vi "GetScanCrvInd.vi"(8 "error in (no error)":errorcluster caption="entrée d'erreur (pas d'erreur)", 10 "Curve Ind":i32, 11 "Interface.lvclass":refnum<class "Interface.lvclass">) -> (0 "error out":errorcluster caption="sortie d'erreur", 2 "Curves Index":i32[](array[numeric]), 3 "Interface.lvclass Out":refnum<class "Interface.lvclass">)   [LabVIEW 2019, in "Interface.lvclass"]
uses:
  Interface.lvclass
  Interface.lvclass/Interface.ctl
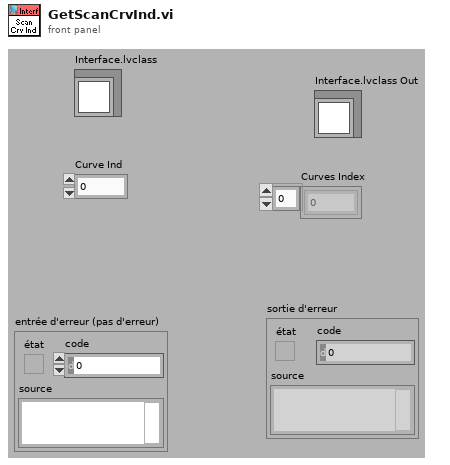
[diagram p1: front panel]
types:
  T1 = typedef "Interface.lvclass/CurveSetup.ctl" = cluster{"CurveName":string, "YParam":string, "XParam":string, "ZParam ":string, "GroupName":string, "LinWdth":u8, "PntCol":u32, "LinCol":u32, "LablFor":u8, "XScale":u32, "YScale":u32, "Interpol":u8, "DisplayName":string, "FillType":i16, "LineStyle":u8, "PntStyle":u8, "BarTyp":u8, "GraphIndex":i32, "Visible":bool, "XScaleName":string, "YScaleName":string, "XYGraph_Ref":refnum<vi>, "Data Only":bool, "DataQ Ref":refnum<queue>, "XParQ Ref":refnum<queue>, "XParamInd":i32, "ScanInd":i32, "File Path":path}
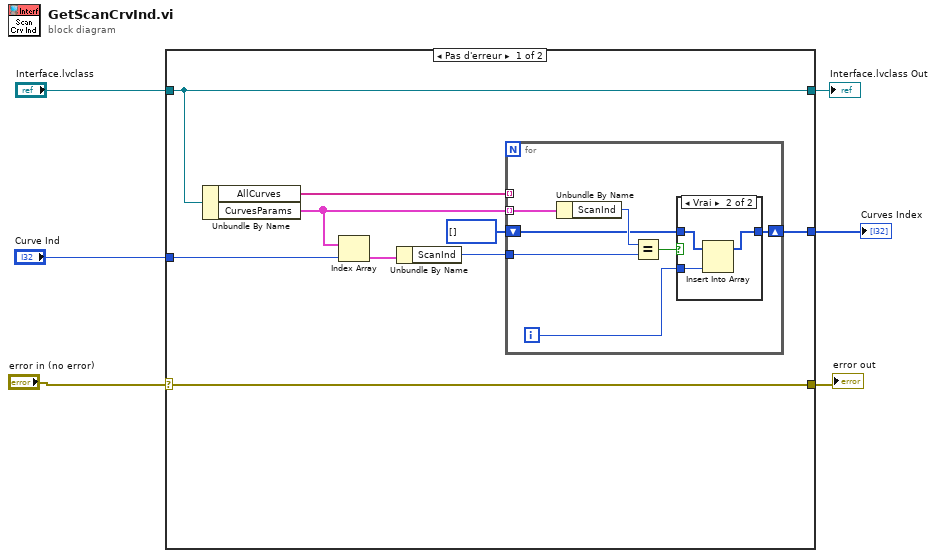
[diagram p0: block diagram]
diagram:
  n1 = case shown="Pas d'erreur" "error in (no error)" {
    selector: "error in (no error)" -> [w15 w28]
    tunnel: [w15 w28] -> w5
    tunnel: [w14 w27] -> w4
    tunnel: "Interface.lvclass" -> [w14 w27]
    tunnel: [w12 _] -> w2
    tunnel: "Curve Ind" -> [w10 _]
    frame No Error {
      n2 = Unbundle By Name(w14) -> ("AllCurves"=w13:string[], "CurvesParams"=w11:T1[])
      n3 = Index Array(array=w11, index=w10) -> (element=w9:T1)
      n4 = Unbundle By Name(w9) -> ("ScanInd"=w8:i32)
      n5 = for {
        tunnel: w13 -> [_] mode=indexing
        tunnel: w11 -> [w22] mode=indexing
        tunnel: w8 -> [w20]
        shift-right: [w17] -> w12
        shift-left: i32[] [] -> [w16]
        i -> [w18]
        n6 = Unbundle By Name(w22) -> ("ScanInd"=w21:i32)
        n7 = Equal?(x=w21, y=w20) -> (x = y?=w19:bool)
        n8 = case shown="Vrai" w19 {
          tunnel: w18 -> [_ w26]
          tunnel: [w23 w25] -> w17
          tunnel: w16 -> [w23 w24]
          frame False {
          }
          frame True {
            n9 = Insert Into Array(array=w24, new element=w26) -> (w25:i32[])  [unwired: 1 in]
          }
        }
      }
    }
    frame Error {
    }
  }
  "Interface.lvclass Out" <- w4
  "error out" <- w5
  "Curves Index" <- w2
